vi "Rename And Move Entire Library.vi"(4 "new folder name (\"\")":string, 5 "project":refnum<vi>, 6 "old folder name (\"\")":string, 7 "new name without extension":string, 8 "error in":errorcluster, 10 "library path":path, 11 "application":refnum<vi>) -> (0 "error out":errorcluster, 2 "new library path":path, 3 "application out":refnum<vi>)   [LabVIEW 2014, in "SequencerActionScript.lvclass"]
doc: "NI Tag Bus Module Framework 1.0.2.36\nNI Systems Engineering"
uses:
  SequencerActionScript.lvclass
  <vilib>/Utility/EditLVLibs/Edit LVLibs.lvlib
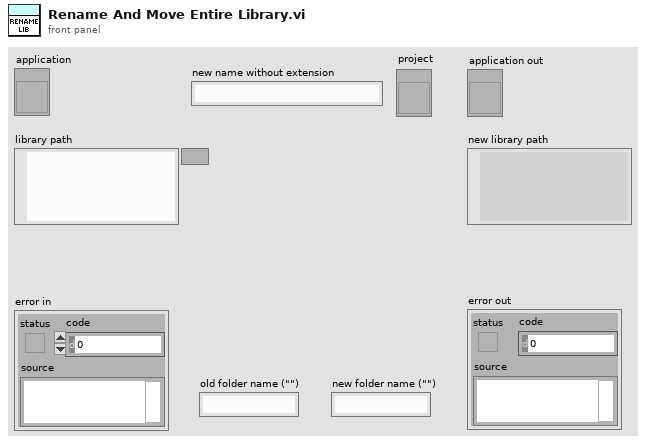
[diagram p1: front panel]
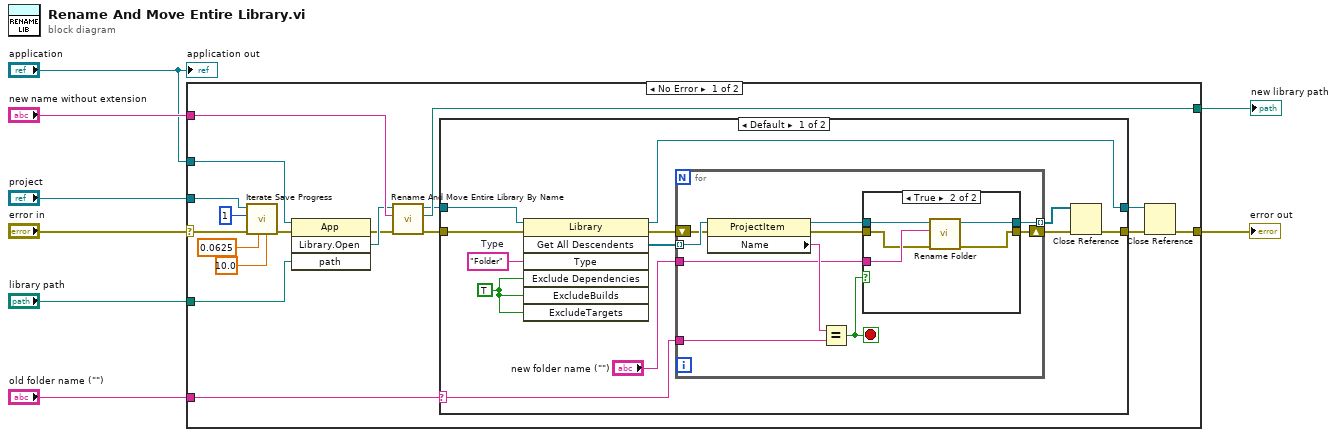
[diagram p0: block diagram]
diagram:
  n1 = case shown="No Error" "error in" {
    selector: "error in" -> [w11 w58]
    tunnel: "application" -> [w26 _]
    tunnel: "library path" -> [w25 _]
    tunnel: "new name without extension" -> [w24 _]
    tunnel: [w21 _] -> w6
    tunnel: [w20 w58] -> w5
    tunnel: "old folder name (\"\")" -> [w19 _]
    tunnel: "project" -> [w9 _]
    frame No Error {
      n2 = call <resource>:"Iterate Save Progress.vi"("Total Iteration Progress"=10.0 ("This Task's Percentage"), "This Task's Percentage"=0.0625, "error in (no error)"=w11, "Total Iterations (this task)"=1, "Project"=w9) -> ("error out"=w10:errorcluster)  [unwired: 6 in]
      n3 = invoke class="App" method="Library.Open"(reference=w26, error in=w10, "path"=w25) -> (error out=w22:errorcluster, "Open Library"=w23:refnum<vi>)  [unwired: 1 in, 2 out]
      n4 = call <vilib>:"Rename And Move Entire Library By Name.vi"("error in (no error)"=w22, "New name without file extension"=w24, "Library ref in"=w23) -> ("error out"=w17:errorcluster, "New Library Path"=w21:path, "Library ref out"=w18:refnum<vi>)  [unwired: 6 in]
      n5 = case shown="Default" w19 {
        selector: w19 -> [w35 _]
        tunnel: w18 -> [w38 w57]
        tunnel: w17 -> [w37 w56]
        tunnel: [w32 w57] -> w16
        tunnel: [w30 w56] -> w15
        frame Default {
          w27 = TRUE
          w28 = "Folder"  # Type
          n6 = invoke class="Library" method="Get All Descendents"(reference=w38, error in=w37, "Type"=w28, "Exclude Dependencies"=w27, "ExcludeBuilds"=w27, "ExcludeTargets"=w27) -> (reference out=w32:refnum<vi>, error out=w33:errorcluster, "All Descendents"=w36:refnum<vi>[])  [unwired: 1 in, 4 out]
          n7 = for {
            tunnel: w36 -> [w48] mode=indexing
            tunnel: w35 -> [w46]
            tunnel: "new folder name (\"\")" -> [w43]
            tunnel: [w39] -> w29 mode=indexing
            shift-right: [w40] -> w31
            shift-left: w33 -> [w42]
            stop <- w45 stop-if-true
            n8 = property class="ProjectItem"(reference=w48, error in=w42) -> (reference out=w44:refnum<vi>, error out=w41:errorcluster, "Name"=w47:string)
            n9 = Equal?(x=w47, y=w46) -> (x = y?=w45:bool)
            n10 = case shown="True" w45 {
              tunnel: w44 -> [w49 w55]
              tunnel: w43 -> [_ w54]
              tunnel: w41 -> [w50 w53]
              tunnel: [w50 w52] -> w40
              tunnel: [w49 w51] -> w39
              frame False {
              }
              frame True {
                n11 = call "Rename Folder.vi"("error in"=w53, "new folder name"=w54, "projectitem in"=w55) -> ("error out"=w52:errorcluster, "projectitem out"=w51:refnum<vi>)  [unwired: 7 in]
              }
            }
          }
          n12 = Close Reference(reference=w29, error in (no error)=w31) -> (error out=w30:errorcluster)
        }
        frame "" {
        }
      }
      n13 = Close Reference(reference=w16, error in (no error)=w15) -> (error out=w20:errorcluster)
    }
    frame Error {
    }
  }
  "error out" <- w5
  "new library path" <- w6
  "application out" <- "application"
